vi "helper_binaryReadAndWrite.vi"() -> ()   [LabVIEW 2021]
uses:
  <vilib>/numeric/Random Number (Range) I64.vi
  <vilib>/numeric/sub_Random U32.vi
panel:
  out "error out 2":errorcluster
  out "data 2":waveform(i16)[](array[waveform])
  out "size(s) 2":i32
  out "size(s)":i32
  out "Array":i32[](array[numeric])
  out "size (in bytes)":i64
  out "data":i16[](array[numeric])
  out "error out":errorcluster
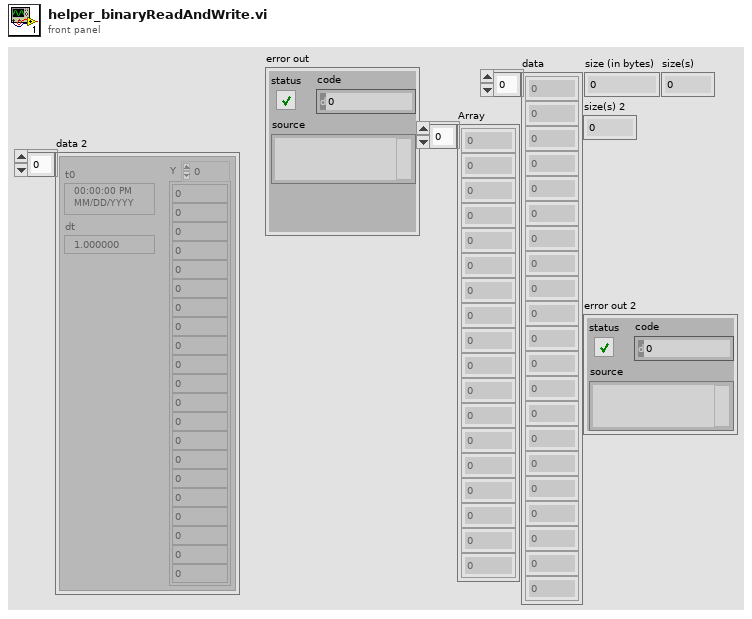
[diagram p1: front panel]
types:
  T1 = enum16{"big-endian, network order", "native, host order", "little-endian"}
  T2 = enum16{"open", "open or create", "create or replace", "create", "open (read-only)"}
  T3 = enum16{"open", "replace", "create", "open or create", "replace or create", "replace or create with confirmation"}
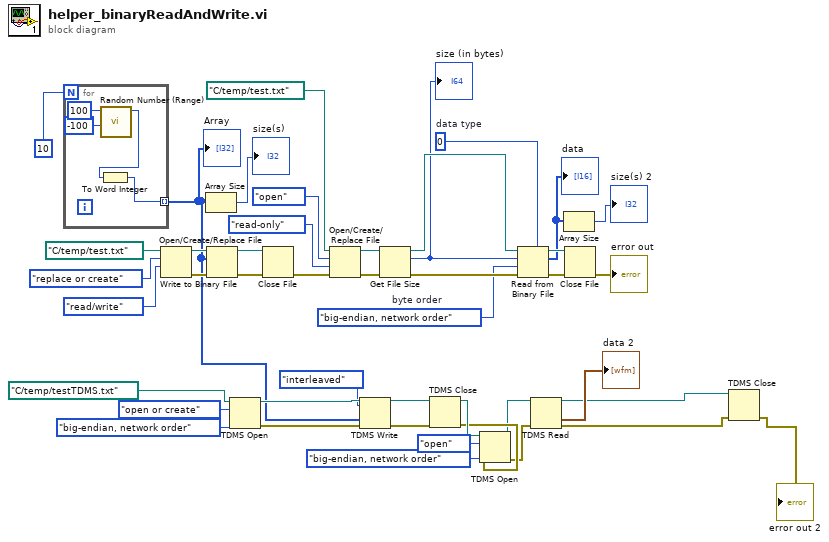
[diagram p0: block diagram]
diagram:
  w28 = T1."big-endian, network order"  # byte order
  w29 = i16 0  # data type
  n1 = for {
    N: 10 -> [_]
    tunnel: [w45] -> w15 mode=indexing
    n2 = call-poly <vilib>:"Random Number (Range).vi"("lower bound (-100)"=i64 -100, "upper bound (100)"=i64 100) -> ("number"=w46:i64)  [unwired: 9 in]
    n3 = To Word Integer(number=w46) -> (16bit integer=w45:i16)
  }
  "Array" <- w15
  n4 = Open/Create/Replace File(file path (use dialog)=path "C:/temp/test.txt", operation (0:open)=T3."replace or create", access (0:read/write)=enum16{"read/write", "read-only", "write-only"}."read/write") -> (refnum out=w40:refnum<file>, error out=w39:errorcluster)  [unwired: 3 in, 1 out]
  n5 = Array Size(array=w15) -> (size(s)=→"size(s)":i32)
  n6 = Write to Binary File(file (use dialog)=w40, data=w15, error in=w39) -> (refnum out=w38:refnum<file>, error out=w37:errorcluster)  [unwired: 3 in, 1 out]
  n7 = TDMS Open(9:T1."big-endian, network order" ("byte order (2:little-endian)"), 10:T2."open or create" ("operation (0:open)"), 11:path "C:/temp/testTDMS.txt" ("file path (use dialog)")) -> (0:w13:errorcluster, 3:w16:refnum<k34>)  [unwired: 4 in]
  n8 = Close File(refnum=w38, error in=w37) -> (error out=w44:errorcluster)  [unwired: 1 out]
  n9 = Open/Create/Replace File(file path (use dialog)=path "C:/temp/test.txt", error in=w44, operation (0:open)=T3."open", access (0:read/write)=enum16{"read/write", "read-only", "write-only"}."read-only") -> (refnum out=w33:refnum<file>, error out=w34:errorcluster)  [unwired: 2 in, 1 out]
  n10 = TDMS Write(0:w16, 1:enum16{"decimated", "interleaved"}."interleaved" ("data layout (0:decimated)"), 9:w15, 11:w13) -> (4:w14:refnum<k34>, 15:w12:errorcluster)  [unwired: 2 in, 2 out]
  n11 = Get File Size(file=w33, error in=w34) -> (refnum out=w31:refnum<file>, size (in bytes)=w20:i64, 0:w32:errorcluster)
  "size (in bytes)" <- w20
  n12 = TDMS Close(8:w12, 11:w14) -> (0:w7:errorcluster, 3:w10:path)
  n13 = TDMS Open(8:w7, 9:T1."big-endian, network order" ("byte order (2:little-endian)"), 10:T2."open" ("operation (0:open)"), 11:w10) -> (0:w6:errorcluster, 3:w5:refnum<k34>)  [unwired: 3 in]
  n14 = Read from Binary File(5:w29, 8:w32, 9:w28, 10:w20, 11:w31) -> (0:w35:errorcluster, 2:w22:i16[], 3:w36:refnum<file>)  [unwired: 1 in, 1 out]
  "data" <- w22
  n15 = TDMS Read(0:w5, 11:w6) -> (4:w3:refnum<k34>, 10:→"data 2":waveform(dbl)[], 15:w2:errorcluster)  [unwired: 6 in, 3 out]
  n16 = Array Size(array=w22) -> (size(s)=→"size(s) 2":i32)
  n17 = Close File(refnum=w36, error in=w35) -> (error out=→"error out":errorcluster)  [unwired: 1 out]
  n18 = TDMS Close(8:w2, 11:w3) -> (0:→"error out 2":errorcluster)  [unwired: 1 out]
